vi "GUI draft.vi"() -> ()   [LabVIEW 2018]
uses:
  Main/Script Step.ctl
  Main/Pump Port.ctl
  Main/Pump Action.ctl
  Main/Drain Valve.ctl
panel:
  in  "Tab Control":enum32{"Main", "Eng", "Script"}(tab)
  in  "Date":string
  in  "Station":string
  in  "Operator":string
  in  "SN4":string
  in  "Cartridge loaded 4":bool
  in  "SN3":string
  in  "Cartridge loaded 3":bool
  in  "SN2":string
  in  "Cartridge loaded 2":bool
  in  "SN1":string
  in  "Cartridge loaded 1":bool
  in  "Time Remaining":string
  in  "Status":string
  in  "Start TW":bool
  out "Progress":u8(slide) scale=0.0..100.0
  in  "Syringe Pump":T3
  in  "Clear Script":bool
  in  "Save Script":bool
  in  "Load Script":bool
  in  "Script Array":T4[](array[typedef])
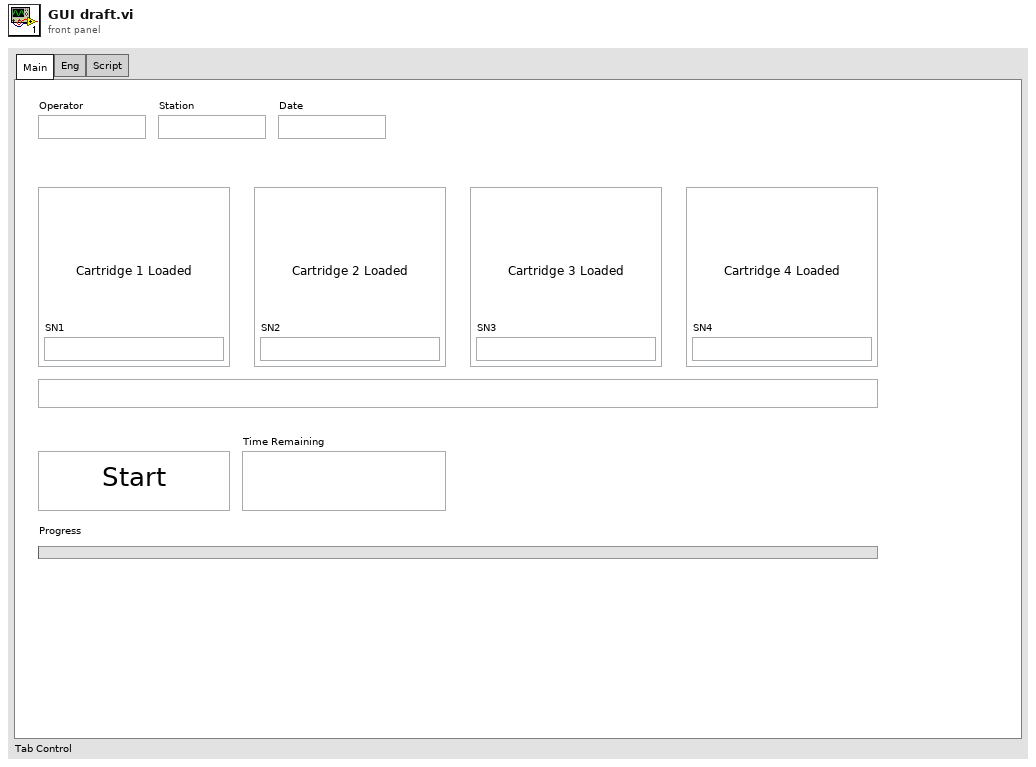
[diagram p1: front panel]
types:
  T1 = typedef "Pump Port.ctl" = enum16{"NaOH", "HCl", "Water", "Methanol", "Detergent", "Vial 1", "Vial 2", "Vial 3", "Vial 4"}
  T2 = typedef "Pump Action.ctl" = enum16{"Draw In", "Draw Out"}
  T3 = cluster{"Port":T1, "Direction":T2, "Amount":dbl, "Pump Start":bool, "Port Set":bool}
  T4 = typedef "Script Step.ctl" = cluster{"Step":dbl, "Step En":bool, "Port":T1, "Direction":T2, "Volume(ul)":dbl, "Rate(ul/s)":dbl, "Pump En":bool, "Drain Valve":T5, "Drain En":bool, "Peristaltic":bool, "Peristaltic En":bool, "Vacuum":bool, "Vacuum En":bool, "Delay(s)":dbl, "Delay En":bool}
  T5 = typedef "Drain Valve.ctl" = enum16{"Vial 1", "Vial 2", "Vial 3", "Vial 4", "Closed"}
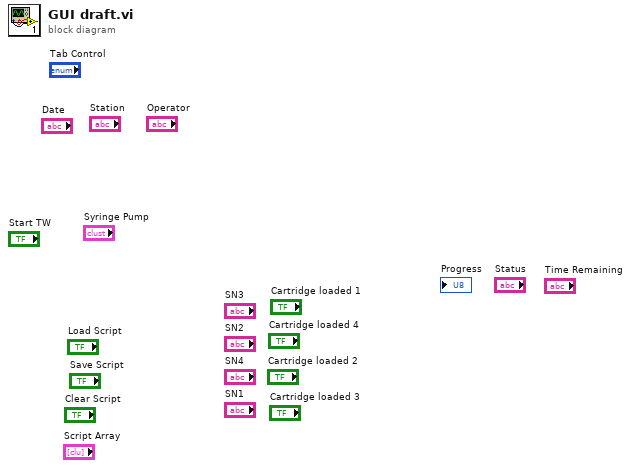
[diagram p0: block diagram]
diagram:
